vi "Main.vi"() -> ()   [LabVIEW 2016]
doc: "The myRIO Project template acquires acceleration data from the onboard accelerometer and displays the changes of acceleration values in a waveform chart."
uses:
  <vilib>/addons/Fuzzy Logic/TypeDefs/FL Input_Output.ctl
  <vilib>/myRIO/Instrument Drivers/Onboard IO/UART/typedef/VISA Configuration.ctl
  <vilib>/myRIO/Instrument Drivers/Onboard IO/DIO/typedefs/DIO Reference.ctl
  <vilib>/myRIO/Common/Instrument Driver Framework/Utilities/typedefs/myRIO Generic Hardware Reference.ctl
  <vilib>/myRIO/Common/Instrument Driver Framework/Utilities/typedefs/Hardware Version Enum.ctl
  <vilib>/myRIO/Common/Instrument Driver Framework/Utilities/typedefs/myRIO v1.0 Reference.ctl
  <vilib>/myRIO/Common/Instrument Driver Framework/Utilities/typedefs/Generic FPGA Reference.ctl
  <vilib>/myRIO/Common/Instrument Driver Framework/myRIO v1.0/DIO/typedefs/DIO Channels List.ctl
  <vilib>/myRIO/Common/Instrument Driver Framework/myRIO v1.0/DIO/typedefs/DIO Channels Enum.ctl
  <vilib>/userdefined/High Color/nirio_resource_hc.ctl
  <vilib>/myRIO/Instrument Drivers/Onboard IO/PWM/typedefs/PWM Reference.ctl
  <vilib>/myRIO/Common/Instrument Driver Framework/myRIO v1.0/PWM/typedefs/PWM Channels Enum.ctl
  <vilib>/myRIO/Instrument Drivers/Onboard IO/PWM/typedefs/PWM Configuration.ctl
  <vilib>/myRIO/Common/Instrument Driver Framework/Utilities/vis/Is FPGA Ref Available.vi
  <vilib>/myRIO/Common/Instrument Driver Framework/myRIO v1.0/PWM/vis/myRIO v1.1 Open PWM.vi
  <vilib>/myRIO/Instrument Drivers/Onboard IO/PWM/vis/Set Duty Cycle and Frequency.vi
  <vilib>/myRIO/Common/Instrument Driver Framework/myRIO v1.0/DIO/vis/myRIO v1.1 Open DIO.vi
  <vilib>/myRIO/Instrument Drivers/Onboard IO/DIO/vis/Write.vi
  <vilib>/myRIO/Common/Instrument Driver Framework/Utilities/vis/Validate Channels.vi
  <vilib>/myRIO/Common/Instrument Driver Framework/myRIO v1.0/PWM/vis/myRIO v1.0 Reserve PWM.vi
  <vilib>/myRIO/Common/Instrument Driver Framework/myRIO v1.0/DIO/vis/myRIO v1.0 Reserve DIO.vi
  <vilib>/myRIO/Common/Instrument Driver Framework/myRIO v1.0/PWM/vis/myRIO v1.0 Build MUX Configuration PWM.vi
  <vilib>/myRIO/Common/Instrument Driver Framework/myRIO v1.0/Resource Manager/vis/myRIO v1.0 Reserve Channel List.vi
  <vilib>/myRIO/Common/Instrument Driver Framework/myRIO v1.0/DIO/vis/myRIO v1.0 Build MUX Configuration DIO.vi
  <vilib>/myRIO/Common/Instrument Driver Framework/myRIO v1.0/Resource Manager/vis/myRIO v1.0 Create Configuration List.vi
  <vilib>/myRIO/Common/Instrument Driver Framework/myRIO v1.0/Resource Manager/vis/myRIO v1.0 Reserve Channel.vi
  <vilib>/myRIO/Common/Instrument Driver Framework/myRIO v1.0/Resource Manager/vis/myRIO v1.0 Unreserve Channel.vi
  <vilib>/myRIO/Common/Instrument Driver Framework/myRIO v1.0/Resource Manager/vis/myRIO v1.0 Build Mutex Name.vi
  <vilib>/Instr/_visa.llb/VISA Configure Serial Port (Instr).vi
  <vilib>/Utility/VariantDataType/GetNumericInfo.vi
  <vilib>/Utility/error.llb/Error Cluster From Error Code.vi
  <vilib>/myRIO/Common/Instrument Driver Framework/myRIO v1.0/myRIO v1.1 Open.vi
  <vilib>/myRIO/Common/Instrument Driver Framework/Utilities/vis/IO Manager.vi
  <vilib>/myRIO/Common/Instrument Driver Framework/Utilities/vis/Configuration Manager.vi
  <vilib>/myRIO/Common/Instrument Driver Framework/myRIO v1.0/Resource Manager/vis/myRIO v1.0 Configure IO.vi
  <vilib>/myRIO/Common/Instrument Driver Framework/myRIO v1.0/myRIO v1.0 Close.vi
  <vilib>/myRIO/Common/Instrument Driver Framework/myRIO v1.0/DIO/vis/myRIO v1.0 Write DIO.vi
  <vilib>/myRIO/Common/Instrument Driver Framework/myRIO v1.0/PWM/vis/myRIO v1.0 Write PWM.vi
  <vilib>/addons/Fuzzy Logic/FL Fuzzy Controller (MISO).vi
  <vilib>/myRIO/Express VI/Onboard IO/UART/UART Express VI.xnode
  <vilib>/express/express arith-compare/Formula/XNode/ExpressFormulaBlockNode.xnode
  <vilib>/myRIO/Express VI/Onboard IO/DO/DO Express VI.xnode
  <vilib>/myRIO/Instrument Drivers/Onboard IO/DIO/vis/myRIO DIO Open.xnode
  <vilib>/myRIO/Express VI/Onboard IO/PWM/PWM Express VI.xnode
  <vilib>/myRIO/Instrument Drivers/Onboard IO/PWM/vis/myRIO PWM Open.xnode
  <vilib>/myRIO/Instrument Drivers/Onboard IO/UART/UART.lvlib
  <vilib>/myRIO/Instrument Drivers/Onboard IO/PWM/PWM.lvlib
  <vilib>/myRIO/Instrument Drivers/Onboard IO/DIO/DIO.lvlib
  <vilib>/addons/Fuzzy Logic/NI_Fuzzy_Logic_API.lvlib
panel:
  in  "Ayman":dbl(slide) scale=0.63..0.7
  in  "Manual PWM":dbl
  out "size(s)":i32
  out "In":dbl
  out "Distance Array":dbl[](array[numeric])
  in  "Stop Button 2":bool
  out "PWM Array":dbl[](array[numeric])
  in  "variable index":i32
  out "membership functions plot":cluster{cluster{"Xi":dbl, "Yi":dbl}[]}[](graph)
  out "Distance fg":dbl
  out "number 2":dbl
  out "number":dbl
  out "double precision float":dbl
  out "coerced(x)":dbl
  out "In Range?":bool
  in  "Fuzzy/Manual":bool
  out "cm/s":dbl
  out "rule-invoked value?":bool
  out "error out":errorcluster
  out "output value":dbl
  out "error":i32
  in  "desired height":i32(slide) scale=0.0..100.0
  in  "C/DIO2 (DIO2)":bool
  in  "C/DIO1 (DIO1)":bool
  out "velocity":string
  in  "Stop Button":bool
  out "Distance":string
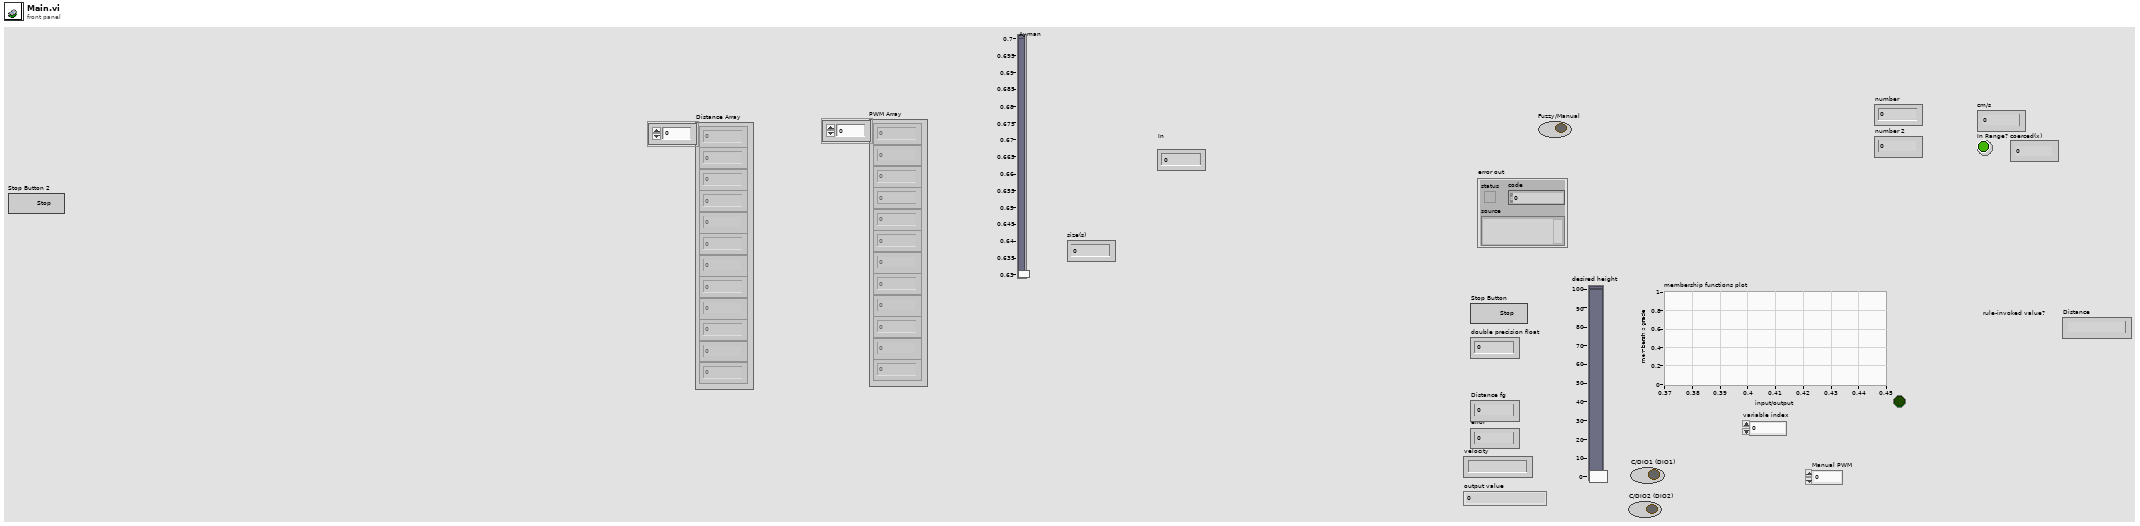
[diagram p1: front panel]
types:
  T1 = typedef "NI_Fuzzy_Logic_API.lvlib/FL System.ctl" = cluster{"input variables":T2[], "output variables":T2[], "rules":T5[], "defuzzification method":T11, "description":string, "user MF interpolating polynomials":T12[]}
  T2 = typedef "NI_Fuzzy_Logic_API.lvlib/FL Variable.ctl" = cluster{"name":string, "range":dbl[], "MFs":T3[]}
  T3 = typedef "NI_Fuzzy_Logic_API.lvlib/FL Membership Function.ctl" = cluster{"name":string, "shape":T4, "points":dbl[], "color":u32, "user-defined shape index":i32}
  T4 = typedef "NI_Fuzzy_Logic_API.lvlib/FL Membership Function Shape.ctl" = u16
  T5 = typedef "NI_Fuzzy_Logic_API.lvlib/FL Rule.ctl" = cluster{"antecedents":T6[], "antecedent connective":T8, "consequents":T9[], "consequent implication":T10, "degree of support":dbl}
  T6 = typedef "NI_Fuzzy_Logic_API.lvlib/FL Antecedent.ctl" = cluster{"Var Index":i32, "MF Index":i32, "Cond":T7}
  T7 = typedef "NI_Fuzzy_Logic_API.lvlib/FL Modifier.ctl" = u16
  T8 = typedef "NI_Fuzzy_Logic_API.lvlib/FL Antecedent Connective.ctl" = u16
  T9 = typedef "NI_Fuzzy_Logic_API.lvlib/FL Consequent.ctl" = cluster{"Var Index":i32, "MF Index":i32, "Cond":T7}
  T10 = typedef "NI_Fuzzy_Logic_API.lvlib/FL Consequent Implication.ctl" = u16
  T11 = typedef "NI_Fuzzy_Logic_API.lvlib/FL Defuzzification.ctl" = u16
  T12 = typedef "NI_Fuzzy_Logic_API.lvlib/FL Interpolating polynomials.ctl" = cluster{"X":dbl[], "Y":dbl[], "Y(x) coeff":dbl[][], "X(y) coeff":dbl[][], "Area(y) coeff":dbl[][], "coa_x(y) coeff":dbl[][]}
  T13 = typedef "DIO.lvlib/DIO Reference.ctl" = cluster{"myRIO Reference":T14, "DIO Channels List":T18}
  T14 = typedef "myRIO Generic Hardware Reference.ctl" = cluster{"myRIO Model":T15, "myRIO Hardware Reference":T16}
  T15 = typedef "Hardware Version Enum.ctl" = enum16{"Unknown", "myRIO-1900", "myRIO-1950", "roboRIO", "NI ELVIS RIO CM"}
  T16 = typedef "myRIO v1.0 Reference.ctl" = cluster{"Generic FPGA Reference":T17, "Allow multiple opens":bool}
  T17 = typedef "Generic FPGA Reference.ctl" = refnum<k20>
  T18 = typedef "DIO Channels List.ctl" = T19[]
  T19 = typedef "DIO Channels Enum.ctl" = enum16{"Not Connected", "C/DIO0", "C/DIO1", "C/DIO2", "C/DIO3", "C/DIO4", "C/DIO5", "C/DIO6", "C/DIO7", "A/DIO0", "A/DIO1", "A/DIO2", "A/DIO3", "A/DIO4", "A/DIO5", "A/DIO6", "A/DIO7", "A/DIO8", "A/DIO9", "A/DIO10", "A/DIO11", "A/DIO12", "A/DIO13", "A/DIO14", "A/DIO15", "B/DIO0", "B/DIO1", "B/DIO2", "B/DIO3", "B/DIO4", "B/DIO5", "B/DIO6", "B/DIO7", "B/DIO8", "B/DIO9", "B/DIO10", "B/DIO11", "B/DIO12", "B/DIO13", "B/DIO14", "B/DIO15", "LED0", "LED1", "LED2", "LED3", "Button0", "DIO/DIO0", "DIO/DIO1", "DIO/DIO2", "DIO/DIO3", "DIO/DIO4", "DIO/DIO5", "DIO/DIO6", "DIO/DIO7", "DIO/DIO8", "DIO/DIO9", "SPI/CS0", "SPI/CS1", "SPI/CS2", "SPI/CS3", "LED RADIO (Green)", "LED RADIO (Red)", "LED COMM (Green)", "LED COMM (Red)", "LED MODE (Green)", "LED MODE (Red)"}
  T20 = typedef "nirio_resource_hc.ctl" = tag
  T21 = typedef "PWM.lvlib/PWM Reference.ctl" = cluster{"myRIO Reference":T14, "PWM Channels Enum":T22, "PWM Configuration":T23}
  T22 = typedef "PWM Channels Enum.ctl" = enum16{"Not Connected", "C/PWM0", "C/PWM1", "A/PWM0", "A/PWM1", "A/PWM2", "B/PWM0", "B/PWM1", "B/PWM2", "PWM/PWM0", "PWM/PWM1", "PWM/PWM2", "PWM/PWM3", "PWM/PWM4", "PWM/PWM5", "PWM/PWM6", "PWM/PWM7", "PWM/PWM8", "PWM/PWM9"}
  T23 = typedef "PWM.lvlib/PWM Configuration.ctl" = cluster{"Frequency":dbl, "Duty Cycle":dbl}
  T24 = typedef "UART.lvlib/VISA Configuration.ctl" = cluster{"baud rate (9600)":u32, "data bits (8)":u16, "parity (0:none)":enum16{"None", "Odd", "Even", "Mark", "Space"}, "stop bits (10: 1 bit)":u16, "flow control (0:none)":u16, "termination char\n(0xA = '\\n' = LF) ":u8, "Enable Termination\nChar (T)":bool, "timeout (10sec)":u32}
  T25 = typedef "NI_Fuzzy_Logic_API.lvlib/FL Input_Output.ctl" = u16
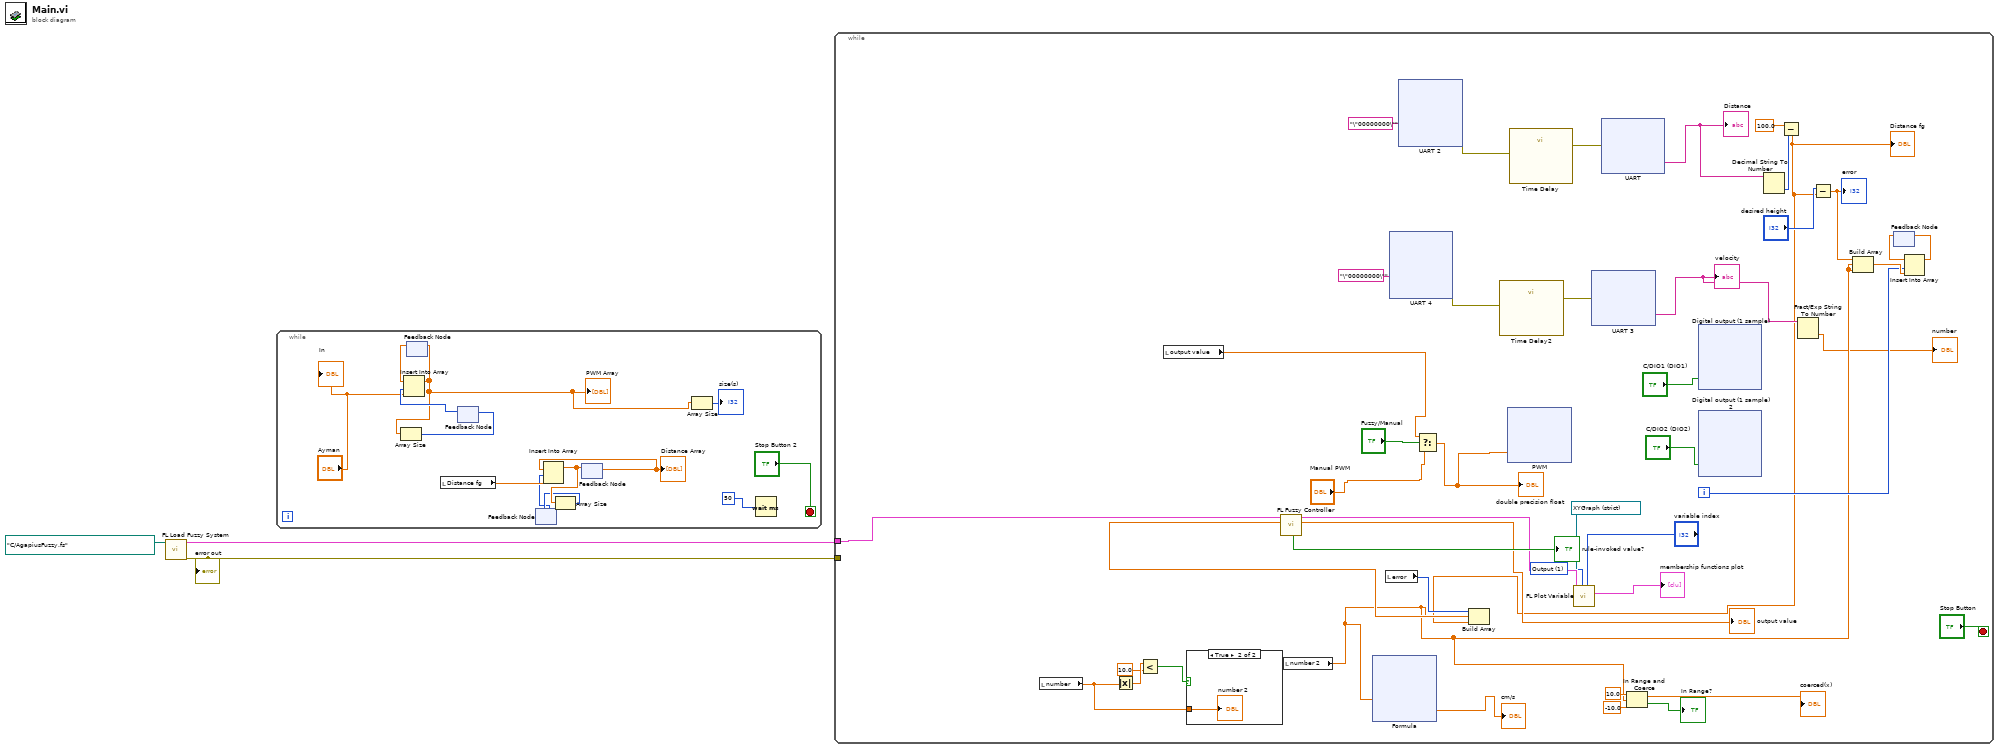
[diagram p0: block diagram]
diagram:
  n1 = call <vilib>:"FL Load Fuzzy System.vi"("file path"=path "C:/AgapiusFuzzy.fs") -> ("error out"=w2:errorcluster, "fuzzy system out"=w3:T1)  [unwired: 9 in]
  "error out" <- w2
  n2 = while {
    stop <- "Stop Button 2" stop-if-true
    n3 = feedback #1() -> (w16:dbl[])  [unwired: 1 in]
    n4 = local read "Distance fg"() -> (w11:dbl)
    n5 = feedback #2() -> (w12:i32)  [unwired: 1 in]
    n6 = Insert Into Array(array=w16, index=w12, new element="Ayman") -> (w6:dbl[])
    "PWM Array" <- w6
    n7 = Array Size(array=w6) -> (size(s)=w13:i32)
    n8 = feedback-in #1(w6) -> ()
    n9 = feedback-in #2(w13) -> ()
    n10 = feedback #3() -> (w7:i32)  [unwired: 1 in]
    n11 = feedback #4() -> (w10:dbl[])  [unwired: 1 in]
    "Distance Array" <- w10
    n12 = Insert Into Array(array=w10, index=w7, new element=w11) -> (w9:dbl[])
    n13 = Array Size(array=w9) -> (size(s)=w8:i32)
    n14 = feedback-in #3(w8) -> ()
    n15 = feedback-in #4(w9) -> ()
    n16 = Array Size(array=w6) -> (size(s)=→"size(s)":i32)
    n17 = Wait (ms)(milliseconds to wait=u32 50) -> ()  [unwired: 1 out]
    "In" <- "Ayman"
  }
  n18 = while {
    tunnel: w3 -> [w35]
    tunnel: w2 -> [_]
    i -> [w43]
    stop <- "Stop Button" stop-if-true
    w22 = T25 1 items=["Input", "Output"] ("input/output")
    n19 = local read "number"() -> (w27:dbl)
    n20 = Absolute Value(x=w27) -> (abs(x)=w30:dbl)
    n21 = Less?(x=w30, y=10.0) -> (x < y?=w31:bool)
    n22 = local read "output value"() -> (w32:dbl)
    n23 = case shown="True" w31 {
      tunnel: w27 -> [_ w62]
      frame False {
      }
      frame True {
        "number 2" <- w62
      }
    }
    n24 = local read "number 2"() -> (w26:dbl)
    n25 = xnode "Formula"("X1"=w26) -> ("Result"=→"cm/s":dbl)  [unwired: 1 in, 1 out]
    n26 = local read "error"() -> (w51:i32)
    n27 = xnode "UART 4"("Characters to Write"="\"00000000\"") -> ("error out"=w56:errorcluster)  [unwired: 1 in, 1 out]
    n28 = xnode "UART 2"("Characters to Write"="\"00000000\"") -> ("error out"=w59:errorcluster)  [unwired: 1 in, 1 out]
    n29 = Select(t=w32, s="Fuzzy/Manual", f="Manual PWM") -> (s? t:f=w17:dbl)
    "double precision float" <- w17
    n30 = call "Time Delay2"("error in (no error)"=w56) -> ("error out"=w55:errorcluster)  [unwired: 10 in]
    n31 = xnode "PWM"("Duty Cycle"=w17) -> ()  [unwired: 1 in, 1 out]
    n32 = call "Time Delay"("error in (no error)"=w59) -> ("error out"=w58:errorcluster)  [unwired: 10 in]
    n33 = xnode "UART 3"("error in (no error)"=w55) -> ("Characters Read"=w29:string)  [unwired: 1 out]
    "velocity" <- w29
    n34 = xnode "UART"("error in (no error)"=w58) -> ("Characters Read"=w52:string)  [unwired: 1 out]
    "Distance" <- w52
    n35 = In Range and Coerce(upper limit=10.0, x=w26, lower limit=-10.0) -> (coerced(x)=→"coerced(x)":dbl, In Range?=→"In Range?":bool)
    n36 = xnode "Digital output (1 sample)"("C/DIO1 (DIO1)"="C/DIO1 (DIO1)") -> ()  [unwired: 1 in, 1 out]
    n37 = xnode "Digital output (1 sample) 2"("C/DIO2 (DIO2)"="C/DIO2 (DIO2)") -> ()  [unwired: 1 in, 1 out]
    n38 = Decimal String To Number(string=w52) -> (number=w48:i32)  [unwired: 2 in, 1 out]
    n39 = Subtract(x=100.0, y=w48) -> (x-y=w25:dbl)
    "Distance fg" <- w25
    n40 = Build Array(w51, w26, w25) -> (w34:dbl[])
    n41 = call-poly <vilib>:"FL Fuzzy Controller.vi"("input values"=w34, "fuzzy system in"=w35) -> ("output value"=→"output value":dbl, "fuzzy system out"=w23:T1, "rule-invoked value?"=→"rule-invoked value?":bool)  [unwired: 5 in, 2 out]
    n42 = call <vilib>:"FL Plot Variable.vi"("variable index"="variable index", "input/output"=w22, "graph refnum"=refnum<vi> refnum, "fuzzy system in"=w23) -> ("membership functions plot"=→"membership functions plot":cluster{cluster{"Xi":dbl, "Yi":dbl}[]}[])  [unwired: 5 in, 2 out]
    n43 = Fract/Exp String To Number(string=w29) -> (number=→"number":dbl)  [unwired: 3 in, 1 out]
    n44 = Subtract(x="desired height", y=w25) -> (x-y=w47:dbl)
    "error" <- w47
    n45 = Build Array(w47, w26, w26) -> (w46:dbl[])
    n46 = feedback #5() -> (w44:dbl[])  [unwired: 1 in]
    n47 = Insert Into Array(array=w44, index=w43, new element=w46) -> (w45:dbl[])
    n48 = feedback-in #5(w45) -> ()
  }
